vi "Config D-A Output.vi"(0 "VISA resource name":refnum<visa-resource-name>, 1 "Outout Format (0: Select)":u16(ring) items=["Select", "Normal", "Integration"], 5 "Channel (1)":u16=1 min=1 max=12 step=1, 7 "Output Item (1: V)":u16(ring)=1 items=["OFF", "V", "A", "W", "VA", "var", "PF", "Phase", "VHz", "AHz", "Wh", "Wh+", "Wh-", "Ah", "Ah+", "Ah-", "Math", "Vpk", "Apk"], 9 "Element (1: Element 1)":u16(ring)=1 items=["", "Element1", "Element2", "Element3", "Sigma"], 11 "error in (no error)":errorcluster) -> (4 "VISA resource name out":refnum<visa-resource-name>, 15 "error out":errorcluster)   [LabVIEW 2016, in "Yokogawa WT200 Series.lvlib"]
doc: "This VI sends the D/A output item to the WT200 Series.\n\nNote : It needs /D4, /D12, /CMP option."
uses:
  Yokogawa WT200 Series.lvlib
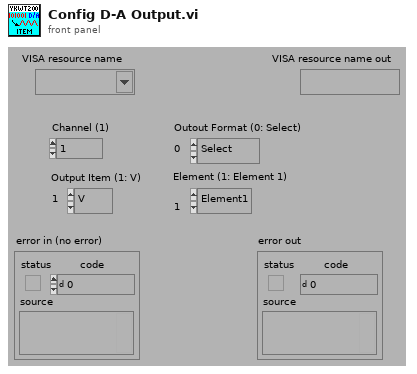
[diagram p1: front panel]
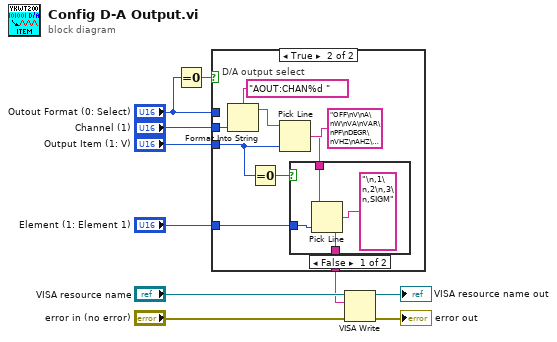
[diagram p0: block diagram]
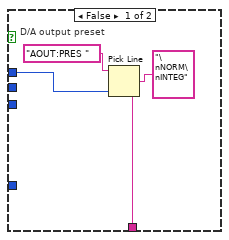
[diagram p2: hidden frame]
diagram:
  n1 = Equal To 0?(x="Outout Format (0: Select)") -> (x = 0?=w4:bool)
  n2 = case shown="True" w4 {
    tunnel: "Output Item (1: V)" -> [_ w23]
    tunnel: "Channel (1)" -> [_ w20]
    tunnel: [w11 w16] -> w2
    tunnel: "Outout Format (0: Select)" -> [w14 _]
    tunnel: "Element (1: Element 1)" -> [_ w15]
    frame False {
      # "D/A output preset"
      n3 = Pick Line(string ("")="AOUT:PRES ", multi-line string="\nNORM\nINTEG", line index=w14) -> (output string=w11:string)
    }
    frame True {
      # "D/A output select"
      n4 = Format Into String(format string="AOUT:CHAN%d ", w20) -> (resulting string=w18:string)  [unwired: 2 in, 1 out]
      n5 = Equal To 0?(x=w23) -> (x = 0?=w22:bool)
      n6 = Pick Line(string ("")=w18, multi-line string="OFF\nV\nA\nW\nVA\nVAR\nPF\nDEGR\nVHZ\nAHZ\nWH\nWHP\nWHM\nAH\nAHP\nAHM\nMATH\nVPK\nAPK", line index=w23) -> (output string=w19:string)
      n7 = case shown="False" w22 {
        tunnel: w19 -> [w26 w28]
        tunnel: [w25 w28] -> w16
        tunnel: w15 -> [w24 _]
        frame False {
          n8 = Pick Line(string ("")=w26, multi-line string="\n,1\n,2\n,3\n,SIGM" ("ÏÙÁ×²Ý•¶Žš—ñ"), line index=w24) -> (output string=w25:string)
        }
        frame True {
        }
      }
    }
  }
  n9 = VISA Write(VISA resource name="VISA resource name", write buffer=w2, error in (no error)="error in (no error)") -> (VISA resource name out=→"VISA resource name out":refnum<visa-resource-name>, error out=→"error out":errorcluster)  [unwired: 1 out]
